vi "FTW-ProjectItemManager-TransactionQueueInfo.vi"(0 "Project Item Manager":refnum<class "FTW-ProjectItemManager.lvclass">, 11 "error in":errorcluster) -> (4 "Project Item Manager out":refnum<class "FTW-ProjectItemManager.lvclass">, 6 "Write Transaction Tags":string[](array[string]), 8 "Remove Transaction Tags":string[](array[string]), 10 "Unapplied Changes?":bool, 15 "error out":errorcluster)   [LabVIEW 2012, in "FTW-ProjectItemManager.lvclass"]
uses:
  FTW-ProjectItemManager.lvclass
  FTW-ProjectItemManager.lvclass/FTW-ProjectItemManager.ctl
panel:
  # "Inputs"
  # "Outputs"
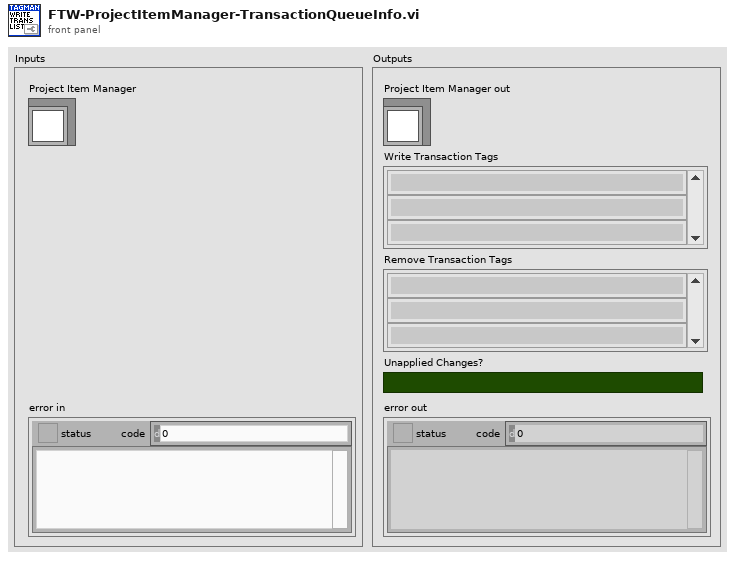
[diagram p1: front panel]
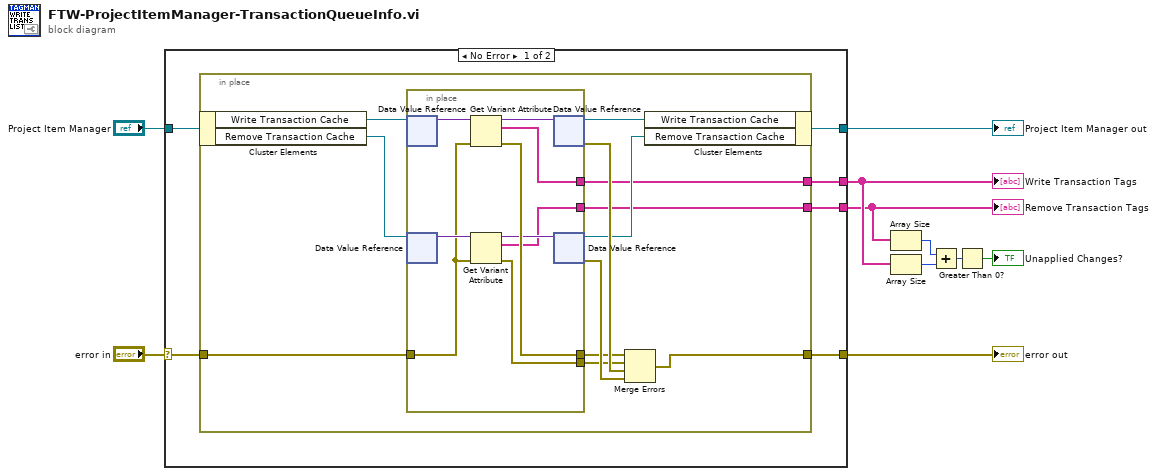
[diagram p0: block diagram]
diagram:
  n1 = case shown="No Error" "error in" {
    selector: "error in" -> [w16 w39]
    tunnel: [w15 w39] -> w10
    tunnel: [w13 w38] -> w8
    tunnel: "Project Item Manager" -> [w14 w38]
    tunnel: [w12 _] -> w6
    tunnel: [w11 _] -> w4
    frame No Error {
      n2 = in-place {
        in-place-border: w16 -> [w26]
        in-place-border: [w22] -> w15
        in-place-border: [w18] -> w12
        in-place-border: [w17] -> w11
        n3 = in-place-cluster #1(w14) -> ("Write Transaction Cache"=w25:refnum<data-value>, "Remove Transaction Cache"=w21:refnum<data-value>)
        n4 = in-place {
          in-place-border: w26 -> [w32]
          in-place-border: [w37] -> w23
          in-place-border: [w34] -> w18
          in-place-border: [w31] -> w20
          in-place-border: [w29] -> w17
          n5 = in-place-dvr #2(w25) -> (w36:variant)  [unwired: 1 out]
          n6 = in-place-dvr #3(w21) -> (w33:variant)  [unwired: 1 out]
          n7 = Get Variant Attribute(Variant=w36, error in=w32) -> (duplicate Variant=w35:variant, names=w34:string[], error out=w37:errorcluster)  [unwired: 2 in, 1 out]
          n8 = Get Variant Attribute(Variant=w33, error in=w32) -> (duplicate Variant=w30:variant, names=w29:string[], error out=w31:errorcluster)  [unwired: 2 in, 1 out]
          n9 = in-place-dvr #2(w35) -> (w24:refnum<data-value>, w28:errorcluster)
          n10 = in-place-dvr #3(w30) -> (w19:refnum<data-value>, w27:errorcluster)
        }
        n11 = Merge Errors(w23, w20, w28, w27) -> (w22:errorcluster)
        n12 = in-place-cluster #1("Write Transaction Cache"=w24, "Remove Transaction Cache"=w19) -> (w13:refnum<class "FTW-ProjectItemManager.lvclass">)
      }
    }
    frame Error {
    }
  }
  "error out" <- w10
  "Project Item Manager out" <- w8
  "Write Transaction Tags" <- w6
  "Remove Transaction Tags" <- w4
  n13 = Array Size(array=w4) -> (size(s)=w3:i32)
  n14 = Array Size(array=w6) -> (size(s)=w2:i32)
  n15 = Add(x=w3, y=w2) -> (x+y=w1:i32)
  n16 = Greater Than 0?(x=w1) -> (x > 0?=→"Unapplied Changes?":bool)
